vi "UE9 DAC Function Generator.vi"() -> ()   [LabVIEW 2021]
uses:
  <vilib>/measure/NI_MABase.lvlib
panel:
  in  "Update Interval (ms)":u32=20
  out "Error":string
  in  "Function":u16(ring) items=["Sine Wave", "Triangle Wave", "Square Wave", "Sawtooth Wave"]
  in  "Min Voltage":dbl=0.5 min=0.0 max=5.0 step=0.1 format="%.2f"
  in  "Max Voltage":dbl=4.5 min=0.0 max=5.0 step=0.1 format="%.2f"
  out "Waveform Chart":dbl(graph)
  in  "Frequency (Hz)":dbl=1.0 step=0.1 format="%.3f"
  in  "Stop":bool
  # "Updates DAC0 at the specified update interval in order to build time series waveforms.  The\nupdate interval is set to 20 ms by default, but can be set lower based on the execution times\ndiscussed in Section 3.1 of the UE9 User's Guide.  Uses the first found USB UE9.\n\nWith a software timed application such as this, you might be able to reduce timing jitter (caused\nby the operating system) by increasing the priority of this process (labview.exe) in Windows\nTask Manager."
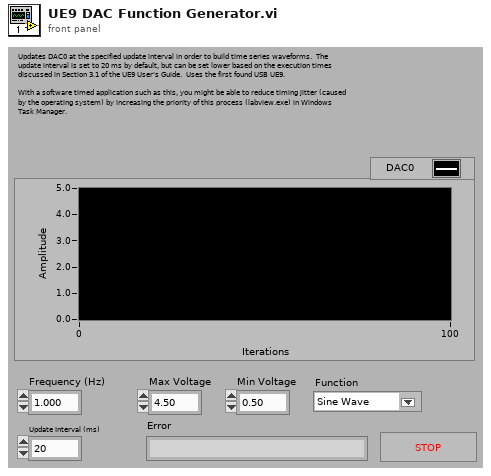
[diagram p1: front panel]
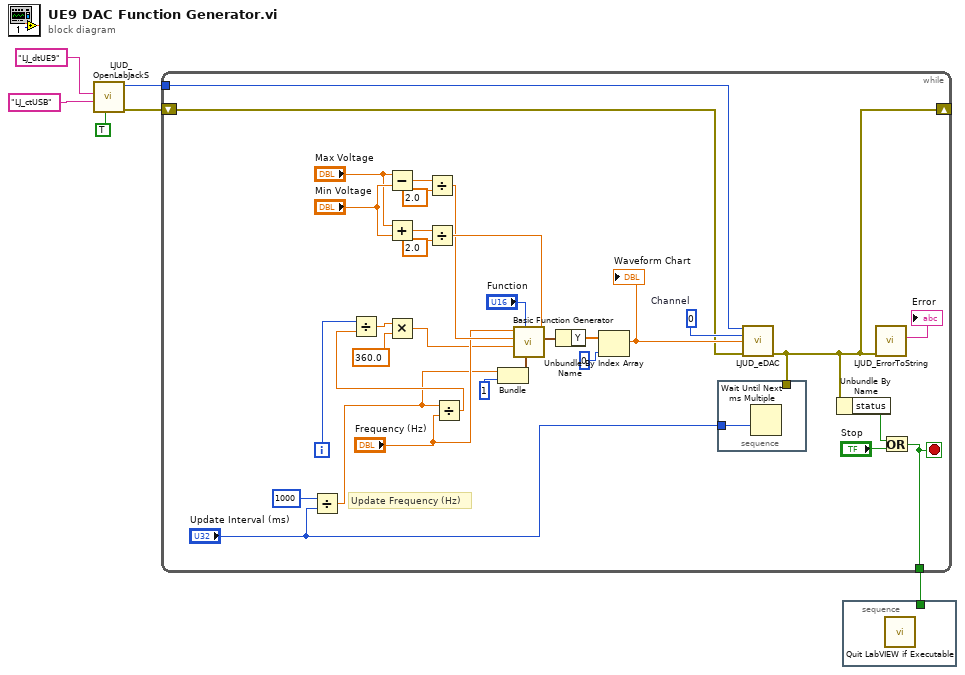
[diagram p0: block diagram]
diagram:
  n1 = call "LJUD_OpenLabJackS.vi"("FirstFound"=TRUE, "ConnectionType"="LJ_ctUSB", "DeviceType"="LJ_dtUE9") -> ("error out"=w2:errorcluster, "Handle"=w1:i32)  [unwired: 6 in, 1 out]
  n2 = while {
    tunnel: w1 -> [w10]
    shift-left: w2 -> [w12]
    shift-right: [w11] -> _
    tunnel: [w14] -> w6
    i -> [w38]
    stop <- w14 stop-if-true
    w13 = 0  # Channel
    # "Update Frequency (Hz)"
    n3 = Divide(x=u32 1000, y="Update Interval (ms)") -> (x/y=w8:dbl)
    n4 = Subtract(x="Max Voltage", y="Min Voltage") -> (x-y=w35:dbl)
    n5 = Add(x="Max Voltage", y="Min Voltage") -> (x+y=w32:dbl)
    n6 = Divide(x=w35, y=2.0) -> (x/y=w27:dbl)
    n7 = Divide(x=w32, y=2.0) -> (x/y=w28:dbl)
    n8 = Divide(x=w8, y="Frequency (Hz)") -> (x/y=w37:dbl)
    n9 = Divide(x=w38, y=w37) -> (x/y=w36:dbl)
    n10 = Multiply(x=w36, y=360.0) -> (x*y=w24:dbl)
    n11 = Bundle(w8, 1) -> (w22:cluster{dbl, i32})  [unwired: 1 in]
    n12 = call <vilib>:"Basic Function Generator.vi"("offset"=w28, "sampling info"=w22, "signal type"="Function", "phase"=w24, "amplitude"=w27, "frequency"="Frequency (Hz)") -> ("signal out"=w21:waveform(dbl))  [unwired: 3 in, 2 out]
    n13 = Unbundle By Name(w21) -> ("Y"=w20:dbl[])
    n14 = Index Array(array=w20, index=0 ("Index")) -> (element=w18:dbl)
    "Waveform Chart" <- w18
    n15 = call "LJUD_eDAC.vi"("Handle In"=w10, "Channel"=w13, "Voltage"=w18, "error in"=w12) -> ("error out"=w11:errorcluster)  [unwired: 10 in, 1 out]
    n16 = stacked-sequence {
      tunnel: "Update Interval (ms)" -> [w39]
      tunnel: w11 -> [_]
      frame #0 {
        n17 = Wait Until Next ms Multiple(millisecond multiple=w39) -> ()  [unwired: 1 out]
      }
    }
    n18 = Unbundle By Name(w11) -> ("status"=w15:bool)
    n19 = call "LJUD_ErrorToString.vi"("error in"=w11) -> ("String"=→"Error":string)  [unwired: 10 in]
    n20 = Or(x=w15, y="Stop") -> (x .or. y?=w14:bool)
  }
  n21 = stacked-sequence {
    tunnel: w6 -> [_]
    frame #0 {
      n22 = call "Quit LabVIEW if Executable.vi"() -> ()  [unwired: 1 in]
    }
  }
